vi "ValueToRecord.vi"(8 "error in (no error)":errorcluster, 11 "Value":string) -> (0 "error out":errorcluster)   [LabVIEW 2018, in "Testing UI 1.lvlib"]
doc: "This subVI enqueues the named action in to the communications queue along with the input data."
uses:
  Testing UI 1.lvlib
  Private Controls/Module Action.ctl
  Private Controls/Module Data.ctl
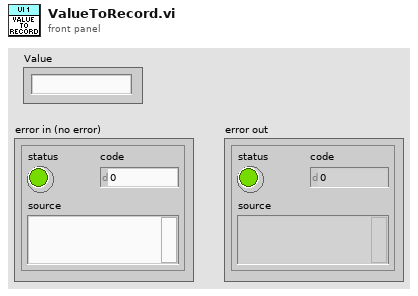
[diagram p1: front panel]
types:
  T1 = typedef "Testing UI 1.lvlib/Module Action.ctl" = enum8{"Init", "Open FP", "Timeout", "New Report Value", "Update Test Info", "Record Data", "Update Report Path", "SetFuelPressure", "Error", "Exit", "Update System Log", "Load APU Setup Data", "Threshold ALERT", "Engine Start Val Change", "Value to Record"}
  T2 = typedef "Testing UI 1.lvlib/Module Data.ctl" = cluster{"Data":variant, "Action":T1}
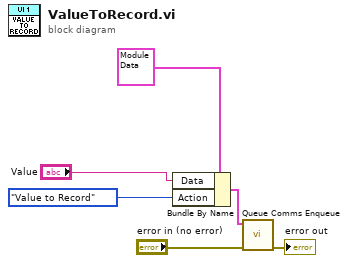
[diagram p0: block diagram]
diagram:
  n1 = Bundle By Name(cluster=T2 {"Data"=variant, "Action"=enum."Init"} ("element"), "Data"="Value", "Action"=Module_Action."Value to Record") -> (w6:T2)
  n2 = call "Queue Comms Enqueue.vi"("error in (no error)"="error in (no error)", "element"=w6) -> ("error out"=→"error out":errorcluster)  [unwired: 9 in]
